vi "State (SubVI).vi"(8 "error in":errorcluster, 11 "Queue in":refnum<queue>) -> (0 "error out":errorcluster, 1 "State":string, 3 "Queue out":refnum<queue>)   [LabVIEW 2017, in "PlayNitrideCameraComponet1010_4.lvlib"]
uses:
  <userlib>/PlayNitrideCameraComponet1010_4/PlayNitrideCameraComponet1010_4.lvlib
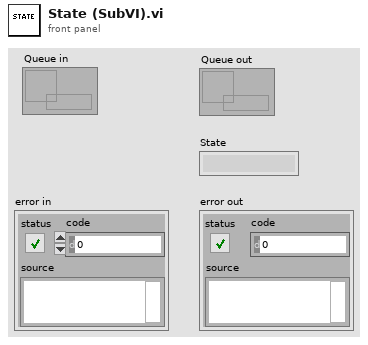
[diagram p1: front panel]
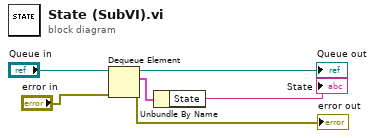
[diagram p0: block diagram]
diagram:
  n1 = Dequeue Element(queue="Queue in", error in (no error)="error in") -> (queue out=→"Queue out":refnum<queue>, element=w3:cluster{"State":string}, error out=→"error out":errorcluster)  [unwired: 1 in, 1 out]
  n2 = Unbundle By Name(w3) -> ("State"=→"State":string)
